vi "Draw All Distances.vi"(10 "CombinedAnchorArray In":refnum<class "Anchor.lvclass">[](array[class])) -> (2 "XY Graph Out":cluster{"x":dbl[], "y":dbl[]}[](graph))   [LabVIEW 2014]
uses:
  Anchor/Anchor.lvclass
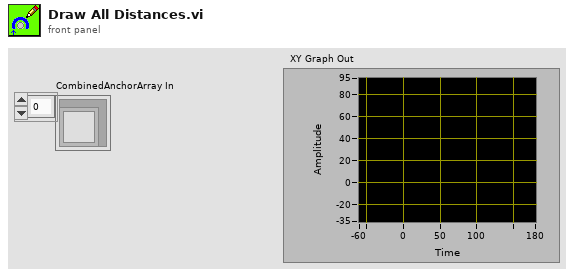
[diagram p1: front panel]
types:
  T1 = cluster{"Tag.lvclass":refnum<class "Tag.lvclass">, "Distance":dbl}[]
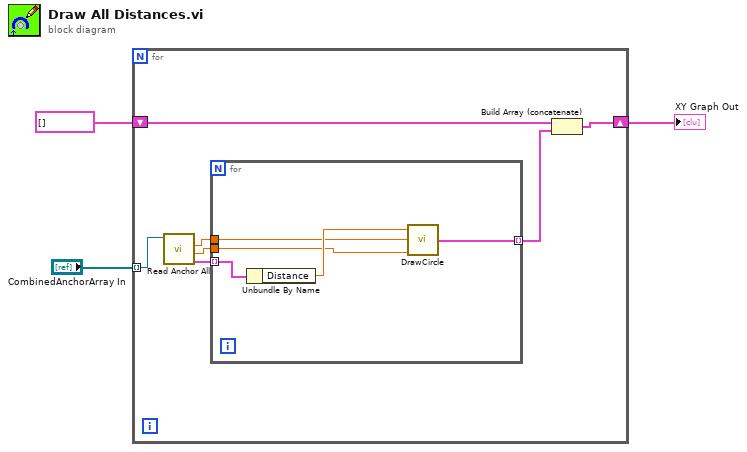
[diagram p0: block diagram]
diagram:
  n1 = for {
    shift-right: [w9] -> w3
    shift-left: cluster{"x":dbl[], "y":dbl[]}[] [] ("XY Graph Out") -> [w10]
    tunnel: "CombinedAnchorArray In" -> [w7] mode=indexing
    n2 = call "Read Anchor All.vi"("Anchor in"=w7) -> ("TagDistanceArray"=w6:T1, "AnchorY"=w5:dbl, "AnchorX"=w4:dbl)  [unwired: 5 in, 3 out]
    n3 = for {
      tunnel: [w15] -> w8 mode=indexing
      tunnel: w6 -> [w14] mode=indexing
      tunnel: w5 -> [w12]
      tunnel: w4 -> [w11]
      n4 = Unbundle By Name(w14) -> ("Distance"=w13:dbl)
      n5 = call "DrawCircle.vi"("y"=w12, "x"=w11, "r"=w13) -> ("XY Graph"=w15:cluster{dbl[], dbl[]})
    }
    n6 = Build Array (concatenate)(w10, w8) -> (w9:cluster{"x":dbl[], "y":dbl[]}[])
  }
  "XY Graph Out" <- w3
